vi "count_string_matches.vi"(0 "String":string="h*el*l*o**w*or*ld", 3 "error in (no error)":errorcluster, 4 "String to Match":string="\\*") -> (7 "Number of matches":i32=7, 10 "error out":errorcluster)   [LabVIEW 2015]
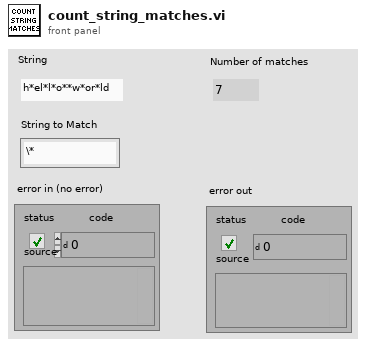
[diagram p1: front panel]
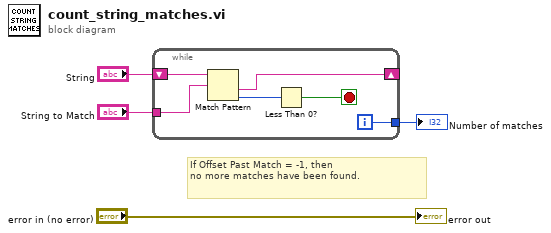
[diagram p0: block diagram]
diagram:
  # "If Offset Past Match = -1, then\nno more matches have been found."
  n1 = while {
    tunnel: [w6] -> w3
    shift-left: "String" -> [w10]
    shift-right: [w9] -> _
    tunnel: "String to Match" -> [w5]
    i -> [w6]
    stop <- w7 stop-if-true
    n2 = Match Pattern(string=w10, regular expression=w5) -> (after substring=w9:string, offset past match=w8:i32)  [unwired: 1 in, 2 out]
    n3 = Less Than 0?(x=w8) -> (x < 0?=w7:bool)
  }
  "Number of matches" <- w3
  "error out" <- "error in (no error)"
